vi "DrawPiece.vi"(8 "error in (no error)":errorcluster, 11 "object in":refnum<class "Piece.lvclass">) -> (0 "error out":errorcluster, 3 "object out":refnum<class "Piece.lvclass">)   [LabVIEW 2020, in "Piece.lvclass"]
uses:
  Piece.lvclass
  Piece.lvclass/Piece.ctl
  typedefs/pieceColor.ctl
  typedefs/pieceType.ctl
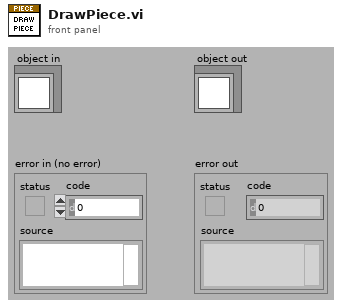
[diagram p1: front panel]
types:
  T1 = typedef "Piece.lvclass/pieceColor.ctl" = enum16{"white", "black"}
  T2 = typedef "Piece.lvclass/pieceType.ctl" = enum16{"K", "Q", "R", "N", "B", "P", "none"}
  T3 = typedef "imagedata.ctl" = cluster{"image type":i32, "image depth":i32, "image":u8[], "mask":u8[], "colors":u32[], "Rectangle":cluster{"left":i16, "top":i16, "right":i16, "bottom":i16}}
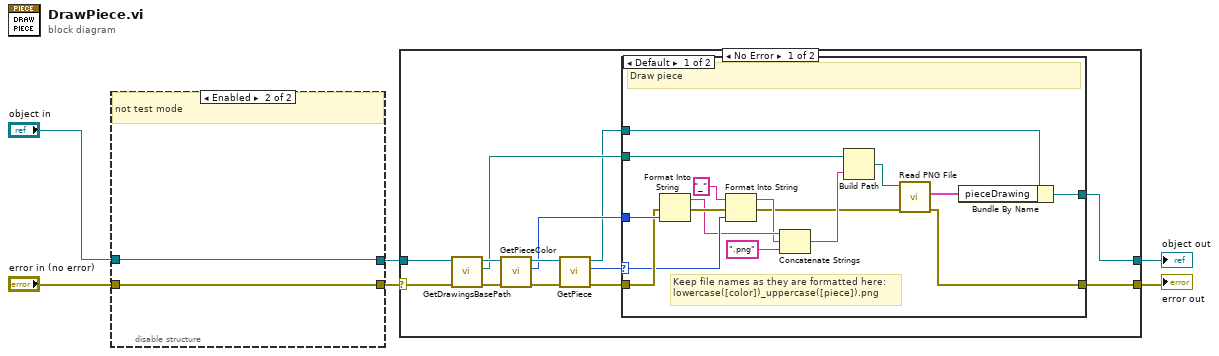
[diagram p0: block diagram]
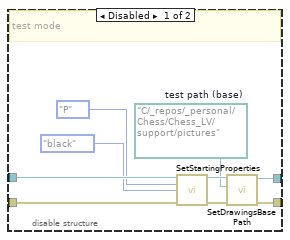
[diagram p4: hidden frame]
diagram:
  n1 = disable-structure shown="Enabled" {
    disable-tunnel: "error in (no error)" -> [w15 w16]
    disable-tunnel: "object in" -> [w13 w17]
    disable-tunnel: [w12 w16] -> w2
    disable-tunnel: [w10 w17] -> w1
    frame Disabled {
      w9 = path "C:/_repos/_personal/Chess/Chess_LV/support/pictures"  # test path (base)
      # "test mode"
      n2 = call "SetStartingProperties.vi"("object in"=w13, "pieceColor"=pieceType."P" ("piece"), "startingSquare"=pieceColor."black" ("pieceColor"), "error in (no error)"=w15) -> ("object out"=w11:refnum<class "Piece.lvclass">, "error out"=w14:errorcluster)  [unwired: 10 in]
      n3 = call "SetDrawingsBasePath.vi"("error in (no error)"=w14, "drawingsBasePath"=w9, "object in"=w11) -> ("error out"=w12:errorcluster, "object out"=w10:refnum<class "Piece.lvclass">)  [unwired: 7 in]
    }
    frame Enabled {
      # "not test mode"
    }
  }
  n4 = case shown="No Error" w2 {
    selector: w2 -> [w30 w50]
    tunnel: [w20 w50] -> w5
    tunnel: [w18 w49] -> w4
    tunnel: w1 -> [w28 w49]
    frame No Error {
      n5 = call "GetDrawingsBasePath.vi"("error in (no error)"=w30, "object in"=w28) -> ("error out"=w29:errorcluster, "drawingsBasePath"=w21:path, "object out"=w26:refnum<class "Piece.lvclass">)  [unwired: 7 in]
      n6 = call "GetPieceColor.vi"("error in (no error)"=w29, "object in"=w26) -> ("error out"=w27:errorcluster, "pieceColor"=w22:T1, "object out"=w25:refnum<class "Piece.lvclass">)  [unwired: 7 in]
      n7 = call "GetPiece.vi"("error in (no error)"=w27, "Piece in"=w25) -> ("error out"=w23:errorcluster, "piece"=w24:T2, "Piece out"=w19:refnum<class "Piece.lvclass">)  [unwired: 5 in, 2 out]
      n8 = case shown="Default" w24 {
        selector: w24 -> [w42 _]
        tunnel: w23 -> [w45 w48]
        tunnel: w22 -> [w46 _]
        tunnel: w21 -> [w38 _]
        tunnel: [w34 w48] -> w20
        tunnel: w19 -> [w33 w47]
        tunnel: [w32 w47] -> w18
        frame Default {
          # "Keep file names as they are formatted here:\nlowercase([color])_uppercase([piece]).png"
          # "Draw piece"
          n9 = Format Into String(error in=w45, w46) -> (resulting string=w41:string, error out=w44:errorcluster)  [unwired: 2 in]
          n10 = Format Into String(initial string="_", error in=w44, w42) -> (resulting string=w40:string, error out=w35:errorcluster)  [unwired: 1 in]
          n11 = Concatenate Strings(w41, w40, ".png" ("string")) -> (w37:string)
          n12 = Build Path(base path=w38, name or relative path=w37) -> (appended path=w36:path)
          n13 = call <vilib>:"Read PNG File.vi"("error in (no error)"=w35, "path to PNG file"=w36) -> ("error out"=w34:errorcluster, "image data"=w31:T3)  [unwired: 7 in, 1 out]
          n14 = Bundle By Name(cluster=w33, "pieceDrawing"=w31) -> (w32:refnum<class "Piece.lvclass">)
        }
        frame "none" {
          # "Do not draw"
        }
      }
    }
    frame Error {
    }
  }
  "error out" <- w5
  "object out" <- w4
